vi "Audio.Generate Multi-Tone Waveform.vi"(6 "DTMF Num":i32, 7 "Amplitude":dbl=1.0, 8 "Tones":T1(array[cluster])=[{"frequency"=1000.0, "amplitude"=1.0, "phase"=0.0}], 9 "Type":enum16{"User Specified", "DTMF"}(ring), 10 "Sample Rate":dbl=44100.0, 11 "Dur(s)":dbl=1.0) -> (1 "Tones Out":T1(array[cluster])=[{"frequency"=1000.0, "amplitude"=1.0, "phase"=0.0}], 3 "Waveform":waveform(dbl))   [LabVIEW 2018]
uses:
  <vilib>/measure/NI_MABase.lvlib
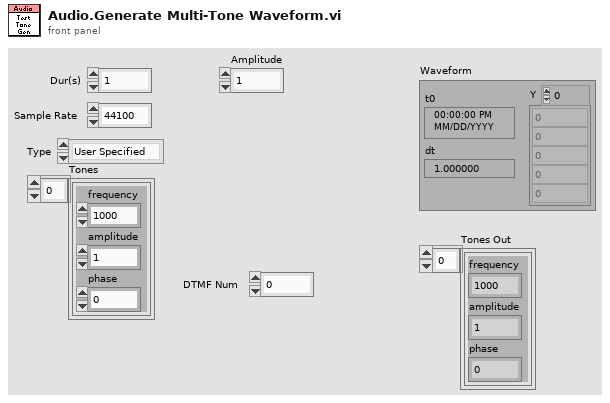
[diagram p1: front panel]
types:
  T1 = cluster{"frequency":dbl, "amplitude":dbl, "phase":dbl}[]
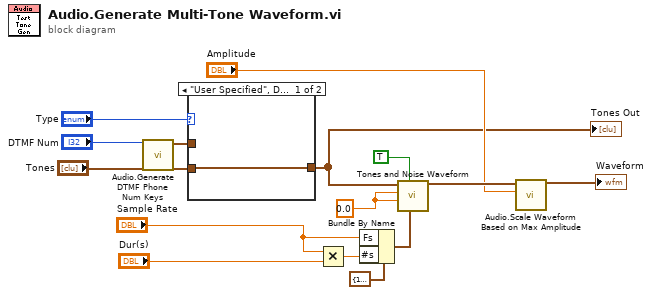
[diagram p0: block diagram]
diagram:
  w15 = 0.0 ("noise (rms)")
  n1 = call "Audio.Generate DTMF Phone Num Keys.vi"("DTMF Num"="DTMF Num") -> ("tones"=w6:T1)  [unwired: 10 in]
  n2 = case shown="\"User Specified\", Default" "Type" {
    tunnel: w6 -> [_ w17]
    tunnel: "Tones" -> [w16 _]
    tunnel: [w16 w17] -> w2
    frame "User Specified", Default {
    }
    frame "DTMF" {
    }
  }
  "Tones Out" <- w2
  n3 = Multiply(x="Sample Rate", y="Dur(s)") -> (x*y=w13:dbl)
  n4 = Bundle By Name(cluster=cluster{"Fs":dbl, "#s":dbl} {"Fs"=1000.0, "#s"=1000.0} ("sampling info"), "Fs"="Sample Rate", "#s"=w13) -> (w12:cluster{"Fs":dbl, "#s":dbl})
  n5 = call <vilib>:"Tones and Noise Waveform.vi"("sampling info"=w12, "reset signal"=TRUE, "offset"=w15, "noise (rms)"=w15, "tones"=w2) -> ("signal out"=w9:waveform(dbl))  [unwired: 5 in, 1 out]
  n6 = call "Audio.Scale Waveform Based on Max Amplitude.vi"("Max Amplitude"="Amplitude", "Wvfrm In"=w9) -> ("Wvfrm Out"=→"Waveform":waveform(dbl))  [unwired: 9 in]
